vi "Last Ack Created Queue.vi"(10 "Queue":refnum<class "Queue.lvclass">, 11 "Last Ack Created Queue in":refnum<class "Last Ack Created Queue.lvclass">) -> (3 "Last Ack Created Queue out":refnum<class "Last Ack Created Queue.lvclass">)   [LabVIEW 2021, in "jettl.lvlib" / "Last Ack Created Queue Msg Strategy.lvlib" / "Last Ack Created Queue.lvclass"]
uses:
  Last Ack Created Queue.lvclass
  Queue/Queue.lvclass
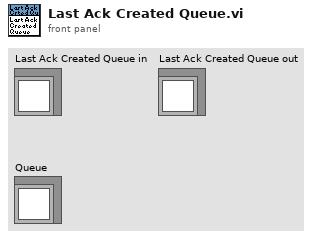
[diagram p1: front panel]
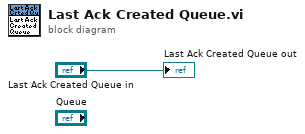
[diagram p0: block diagram]
diagram:
  "Last Ack Created Queue out" <- "Last Ack Created Queue in"
